vi "Invalid ID.vi"(7 "error source vi name":string, 8 "error in (no error)":errorcluster, 10 "id":i32, 11 "Thread Parameters in":refnum<class "Thread Parameters.lvclass">) -> (0 "error out":errorcluster, 3 "Thread Parameters out":refnum<class "Thread Parameters.lvclass">)   [LabVIEW 2017, in "DSF Core.lvlib" / "Thread Parameters.lvclass"]
uses:
  Thread Parameters.lvclass
  Errors.ctl
  <vilib>/NI/Memory Manager/VIs/Source.Write.Scalar.Base10 (I32).vi
  <vilib>/NI/Memory Manager/Static Error Handling.lvlib
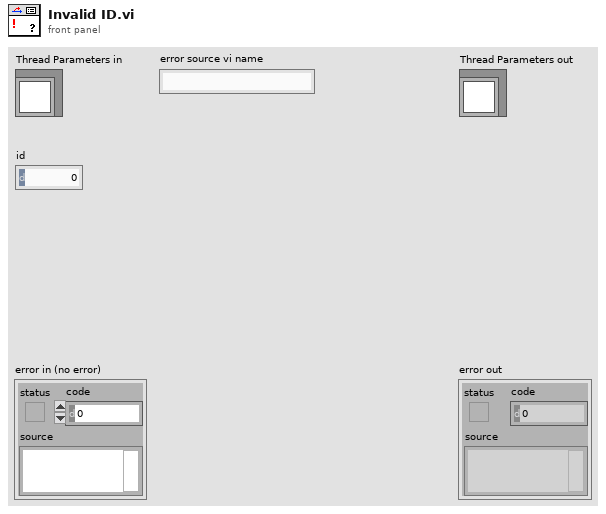
[diagram p1: front panel]
types:
  T1 = typedef "DSF Core.lvlib/Thread Parameters.lvclass/Errors.ctl" = enum16{"Invalid Priority", "Invalid ID"}
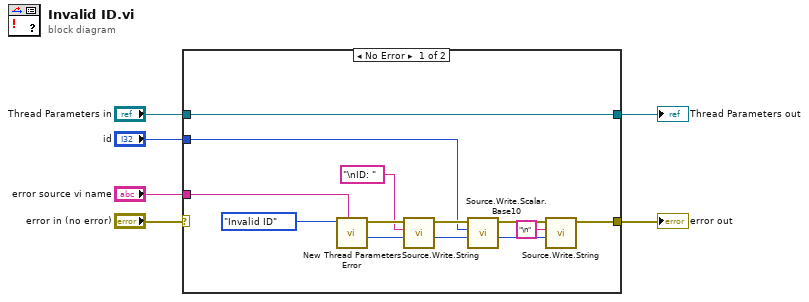
[diagram p0: block diagram]
diagram:
  n1 = case shown="No Error" "error in (no error)" {
    selector: "error in (no error)" -> [_ w20]
    tunnel: "Thread Parameters in" -> [w17 w21]
    tunnel: [w17 w21] -> w4
    tunnel: [w14 w20] -> w3
    tunnel: "error source vi name" -> [w18 _]
    tunnel: "id" -> [w7 _]
    frame No Error {
      n2 = call "New Thread Parameters Error.vi"("error source vi name"=w18, "error"=Errors."Invalid ID") -> ("new offset"=w13:i32, "error out"=w16:errorcluster)  [unwired: 8 in]
      n3 = call <vilib>:"Source.Write.String.vi"("offset"=w13, "string"="\nID: ", "error in"=w16) -> ("new offset"=w12:i32, "error out"=w15:errorcluster)  [unwired: 7 in]
      n4 = call-poly <vilib>:"Source.Write.Scalar.Base10.vi"("offset"=w12, "value"=w7, "error in"=w15) -> ("new offset"=w11:i32, "error out"=w8:errorcluster)  [unwired: 7 in]
      n5 = call <vilib>:"Source.Write.String.vi"("offset"=w11, "string"="\n", "error in"=w8) -> ("error out"=w14:errorcluster)  [unwired: 7 in, 1 out]
    }
    frame Error {
    }
  }
  "error out" <- w3
  "Thread Parameters out" <- w4
